vi "ClientLabViewGrupD.vi"(0 "Missatge a enviar":string(combo)="No enviar res", 1 "Nombre de mostres mitjana":u32=1 min=1 max=9 step=1, 5 "?":bool, 7 "Port":i32=5001, 9 "IP Adress":string="192.168.0.181", 11 "Temps de mostratge":u32=1 min=1 max=20 step=1) -> (2 "Mostra més antiga":dbl, 3 "Temperatura mínima":i32, 4 "Reset":string, 6 "String enviat":string, 8 "String rebut":string, 10 "Error":string, 12 "Status":string, 13 "Mostres Guardades":string, 14 "Temperatura màxima":i32, 15 "Historial de mostres":dbl(graph))   [LabVIEW 2019]
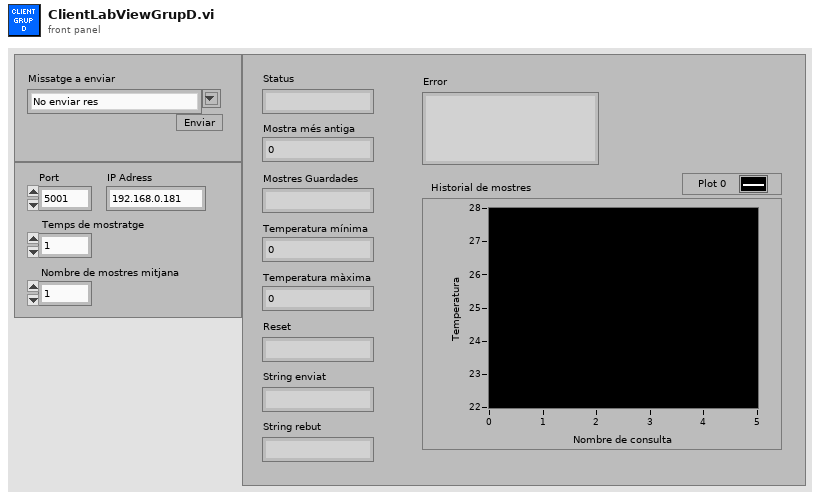
[diagram p1: front panel]
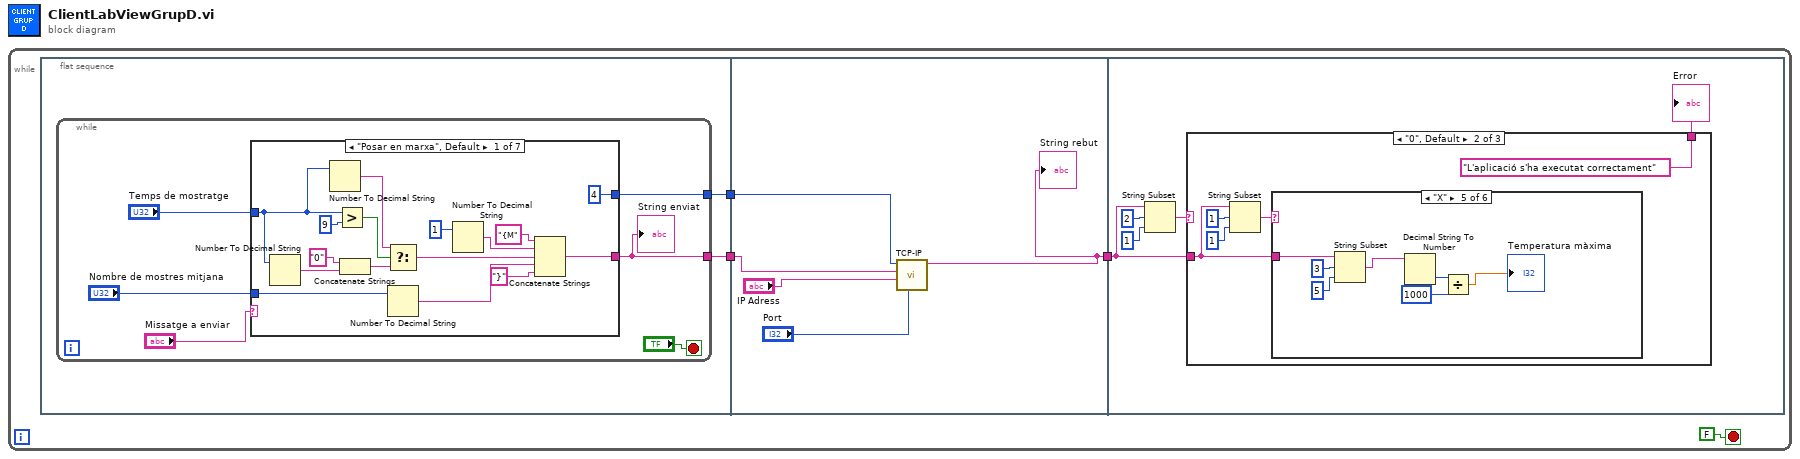
[diagram p0: block diagram]
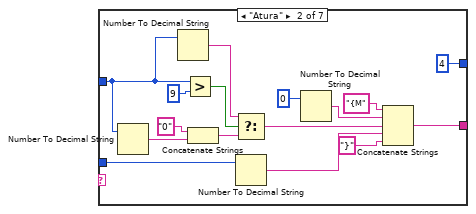
[diagram p2: hidden frame]
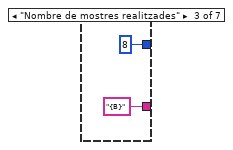
[diagram p3: hidden frame]
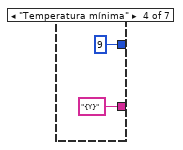
[diagram p4: hidden frame]
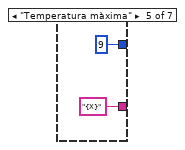
[diagram p5: hidden frame]
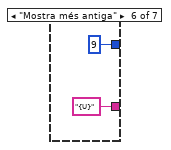
[diagram p6: hidden frame]
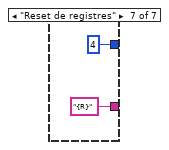
[diagram p7: hidden frame]
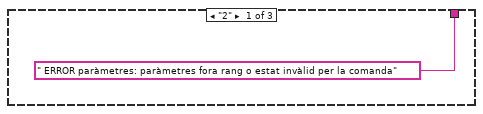
[diagram p8: hidden frame]
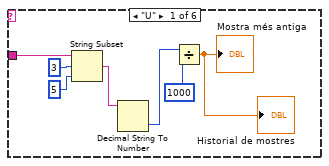
[diagram p9: hidden frame]
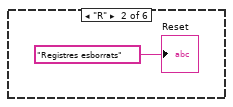
[diagram p10: hidden frame]
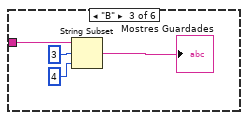
[diagram p11: hidden frame]
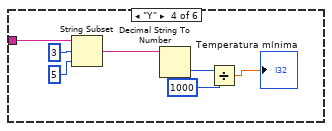
[diagram p12: hidden frame]
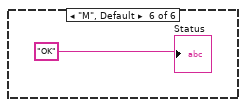
[diagram p13: hidden frame]
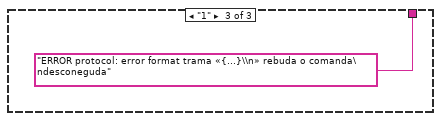
[diagram p14: hidden frame]
diagram:
  n1 = while {
    stop <- FALSE stop-if-true
    n2 = flat-sequence {
      tunnel: [w6] -> w2
      tunnel: [w5] -> w1
      tunnel: [w55] -> w3
      tunnel: w2 -> [w57]
      tunnel: w1 -> [w56]
      tunnel: w3 -> [w61]
      frame #0 {
        n3 = while {
          tunnel: [w7] -> w6
          tunnel: [w8] -> w5
          stop <- "?" stop-if-true
          n4 = case shown="\"Posar en marxa\", Default" "Missatge a enviar" {
            tunnel: [w20 w29 "{B}" "{Y}" "{X}" "{U}" "{R}"] -> w7
            tunnel: [4 4 8 9 9 9 4] -> w8
            tunnel: "Temps de mostratge" -> [w21 w37 _ _ _ _ _]
            tunnel: "Nombre de mostres mitjana" -> [w15 w33 _ _ _ _ _]
            frame "Posar en marxa", Default {
              n5 = Number To Decimal String(number=w21) -> (decimal integer string=w25:string)  [unwired: 1 in]
              n6 = Number To Decimal String(number=w21) -> (decimal integer string=w23:string)  [unwired: 1 in]
              n7 = Greater?(x=w21, y=u32 9) -> (0:w27:bool)
              n8 = Concatenate Strings("0" ("string"), w25) -> (w24:string)
              n9 = Select(t=w23, s=w27, f=w24) -> (s? t:f=w16:string)
              n10 = Number To Decimal String(number=w15) -> (decimal integer string=w14:string)  [unwired: 1 in]
              n11 = Number To Decimal String(number=1 ("input 3")) -> (decimal integer string=w17:string)  [unwired: 1 in]
              n12 = Concatenate Strings("{M", w17, w16, w14, "}") -> (w20:string)
            }
            frame "Atura" {
              n13 = Number To Decimal String(number=w37) -> (decimal integer string=w41:string)  [unwired: 1 in]
              n14 = Number To Decimal String(number=w37) -> (decimal integer string=w39:string)  [unwired: 1 in]
              n15 = Greater?(x=w37, y=u32 9) -> (0:w43:bool)
              n16 = Concatenate Strings("0" ("string"), w41) -> (w40:string)
              n17 = Select(t=w39, s=w43, f=w40) -> (s? t:f=w30:string)
              n18 = Number To Decimal String(number=w33) -> (decimal integer string=w35:string)  [unwired: 1 in]
              n19 = Number To Decimal String(number=0 ("input 3")) -> (decimal integer string=w31:string)  [unwired: 1 in]
              n20 = Concatenate Strings("{M", w31, w30, w35, "}") -> (w29:string)
            }
            frame "Nombre de mostres realitzades" {
            }
            frame "Temperatura mínima" {
            }
            frame "Temperatura màxima" {
            }
            frame "Mostra més antiga" {
            }
            frame "Reset de registres" {
            }
          }
          "String enviat" <- w7
        }
      }
      frame #1 {
        n21 = call "TCP-IP.vi"("Port"="Port", "IP Adress"="IP Adress", "String"=w57, "Numeric"=w56) -> ("data out"=w55:string)  [unwired: 7 in]
        "String rebut" <- w55
      }
      frame #2 {
        n22 = String Subset(string=w61, offset (0)=2, length (rest)=1 ("length (rest)")) -> (substring=w64:string)
        n23 = case shown="\"0\", Default" w64 {
          tunnel: w61 -> [_ w67 _]
          tunnel: [" ERROR paràmetres: paràmetres fora rang o estat invàlid per la comanda" "L'aplicació s'ha executat correctament" "ERROR protocol: error format trama «{...}\\n» rebuda o comanda\ndesconeguda"] -> w60
          frame "2" {
          }
          frame "0", Default {
            n24 = String Subset(string=w67, offset (0)=1, length (rest)=1 ("length (rest)")) -> (substring=w68:string)
            n25 = case shown="\"X\"" w68 {
              tunnel: w67 -> [w77 _ w79 w87 w94 _]
              frame "U" {
                n26 = String Subset(string=w77, offset (0)=3, length (rest)=5 ("length (rest)")) -> (substring=w74:string)
                n27 = Decimal String To Number(string=w74) -> (number=w73:i32)  [unwired: 2 in, 1 out]
                n28 = Divide(x=w73, y=1000) -> (x/y=→"Historial de mostres" →"Mostra més antiga":dbl)
              }
              frame "R" {
                "Reset" <- "Registres esborrats"
              }
              frame "B" {
                n29 = String Subset(string=w79, offset (0)=3, length (rest)=4 ("length (rest)")) -> (substring=→"Mostres Guardades":string)
              }
              frame "Y" {
                n30 = String Subset(string=w87, offset (0)=3, length (rest)=5 ("length (rest)")) -> (substring=w86:string)
                n31 = Decimal String To Number(string=w86) -> (number=w85:i32)  [unwired: 2 in, 1 out]
                n32 = Divide(x=w85, y=1000) -> (x/y=→"Temperatura mínima":dbl)
              }
              frame "X" {
                n33 = String Subset(string=w94, offset (0)=3, length (rest)=5 ("length (rest)")) -> (substring=w93:string)
                n34 = Decimal String To Number(string=w93) -> (number=w92:i32)  [unwired: 2 in, 1 out]
                n35 = Divide(x=w92, y=1000) -> (x/y=→"Temperatura màxima":dbl)
              }
              frame "M", Default {
                "Status" <- "OK"
              }
            }
          }
          frame "1" {
          }
        }
        "Error" <- w60
      }
    }
  }
